vi "Prepare Log.vi"(8 "error in (no error)":errorcluster, 10 "Log":string, 11 "LogHTTPController in":refnum<class "LogHTTPController.lvclass">) -> (0 "error out":errorcluster, 2 "Response":refnum<class "Response.lvclass">, 3 "LogHTTPController out":refnum<class "LogHTTPController.lvclass">)   [LabVIEW 2020, in "VolatusData.lvlib" / "LogHTTPController.lvclass"]
uses:
  LogHTTPController.lvclass
  LogHTTPController.lvclass/LogHTTPController.ctl
  Volatus/MessageQ/MessageQ.lvclass
  lv-http-util/HTTP Utils/Response/Response.lvclass
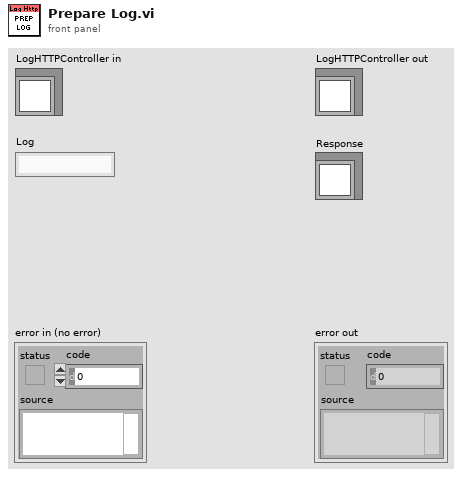
[diagram p1: front panel]
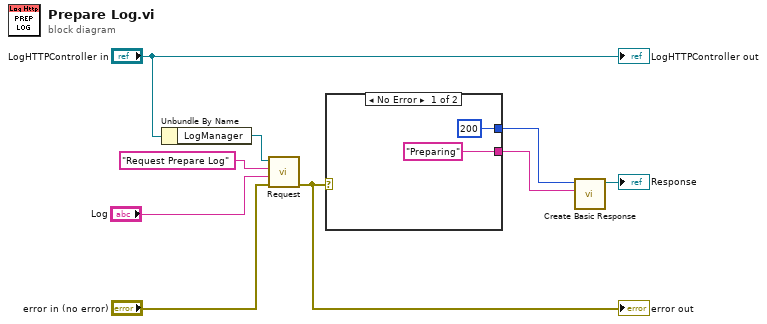
[diagram p0: block diagram]
diagram:
  n1 = Unbundle By Name("LogHTTPController in") -> ("LogManager"=w8:refnum<class "MessageQ.lvclass">)
  n2 = call "Request.vi"("error in (no error)"="error in (no error)", "Data"="Log", "ID"="Request Prepare Log", "MessageQ in"=w8) -> ("error out"=w4:errorcluster)  [unwired: 5 in, 2 out]
  "error out" <- w4
  n3 = case shown="No Error" w4 {
    tunnel: [u16 200 ("Status Code") _] -> w2
    tunnel: ["Preparing" _] -> w1
    frame No Error {
    }
    frame Error {
    }
  }
  n4 = call "Create Basic Response.vi"("Payload"=w1, "Status Code"=w2) -> ("Response out"=→"Response":refnum<class "Response.lvclass">)  [unwired: 8 in, 1 out]
  "LogHTTPController out" <- "LogHTTPController in"
